vi "Target Environment To Number.vi"(11 "Target (Process)":T1 items=["Process", "User", "Machine"]) -> (3 "Number":i32)   [LabVIEW 2019, in "SLL Environment Variable.lvlib"]
doc: "Convert target environment <B>process, user and machine</B> to corresponding numeric values 0, 1 and 2."
uses:
  SLL Environment Variable.lvlib
  _Typedef/Target Environment Enum.ctl
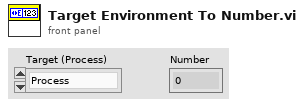
[diagram p1: front panel]
types:
  T1 = typedef "SLL Environment Variable.lvlib/Target Environment Enum.ctl" = i32
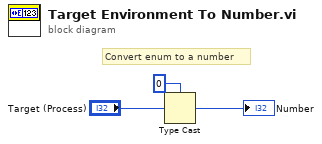
[diagram p0: block diagram]
diagram:
  # "Convert enum to a number"
  n1 = Type Cast(type=0, x="Target (Process)") -> (*(type *) &x=→"Number":i32)
